vi "Adapt Class To Class.vi"() -> ()   [LabVIEW 2020]
doc: "This VI demonstrates a function of the GCraftsman JSON Serialization Toolkit.\n\nLook at the block diagram to see that the 'Adapt to Type' function adapts an object of one class type to an object of another class type. It transfers class private data values to class attributes whose names match. It successfully handles out-of-order and missing or extra class attributes \n\n'Adapt to Type' does not require the classes to have accessor methods \n\nGCraftsman JSON Object Serialization Toolkit\nwww.GCraftsman.com\nCopyright (c) 2017, GCraftsman"
uses:
  library/JKI JSON Object Serialization.lvlib
  Class2/Class2.lvclass
  Class4/Class4.lvclass
panel:
  out "class2.myBool 2":bool
  out "class2.anotherNumber 2":dbl format="%#_13g"
  out "class1.someNumber 2":dbl format="%#_13g"
  in  "class4.myBool 2":bool=TRUE
  in  "class4.someNumber 2":dbl=999.0
  in  "class4.anotherNumber 2":dbl=777.0
  out "class4.myBool":bool
  out "class4.someNumber":dbl
  out "class4.anotherNumber":dbl
  in  "class2.myBool":bool=TRUE
  in  "class2.anotherNumber":dbl=123.0 format="%#_13g"
  in  "class1.someNumber":dbl=456.0 format="%#_13g"
  # "This VI demonstrates a function of the GCraftsman JSON Serialization Toolkit.\n\nLook at the block diagram to see that the 'Adapt to Type' function adapts an object of one class type to an object of another class type.   It transfers class private data values to class attributes whose names match.  It successfully handles out-of-order and missing or extra class attributes \n \nThis example shows that 'Adapt to Type' combines heirarchical class data into a 'flat' class type, and that the 'flat' class data can successfully be distributed to private attributes in a hierarchical class structure.\n\n'Adapt to Type' does not require the classes to have accessor methods"
  # "Class 2 data"
  # "Class 4 data"
  # "parent class data"
  # "child class data"
  # "Class 4 data"
  # "Class 2 data"
  # "parent class data"
  # "child class data"
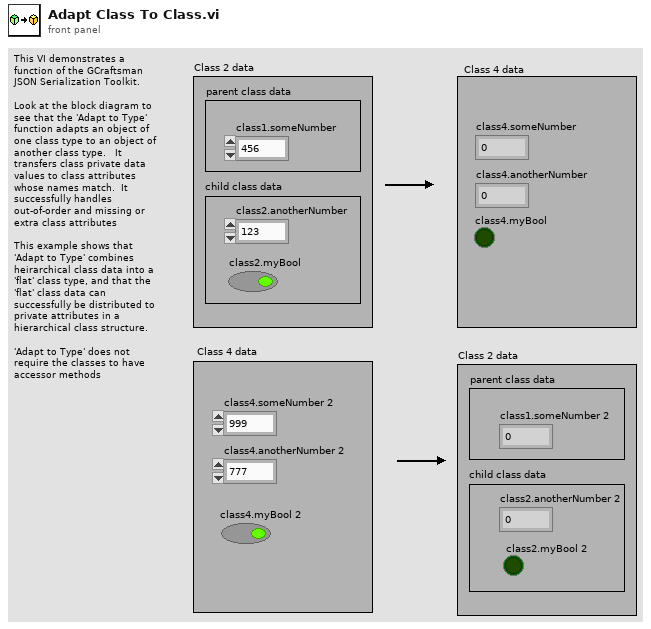
[diagram p1: front panel]
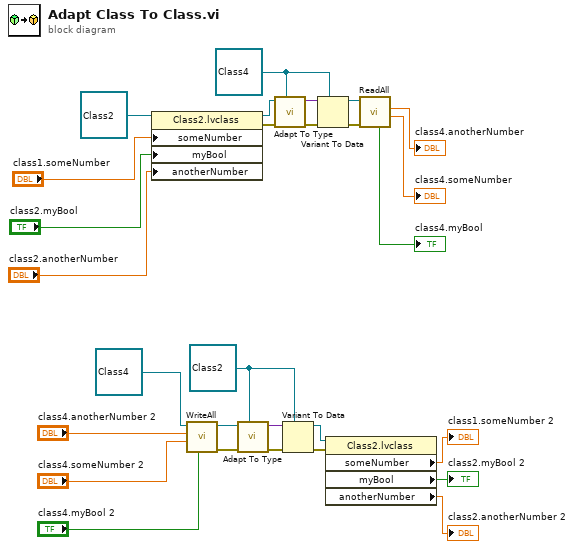
[diagram p0: block diagram]
diagram:
  w9 = refnum<class "Class2.lvclass"> refnum ("Class2.lvclass")
  w21 = refnum<class "Class4.lvclass"> refnum ("Class4.lvclass")
  n1 = property class="Class2.lvclass"(reference=refnum<class "Class2.lvclass"> refnum ("Class2.lvclass"), "someNumber"="class1.someNumber", "myBool"="class2.myBool", "anotherNumber"="class2.anotherNumber") -> (reference out=w22:refnum<class "Class2.lvclass">, error out=w18:errorcluster)  [unwired: 1 in]
  n2 = call "WriteAll.vi"("myBool"="class4.myBool 2", "someNumber"="class4.someNumber 2", "anotherNumber"="class4.anotherNumber 2", "Class4 in"=refnum<class "Class4.lvclass"> refnum ("Class4.lvclass")) -> ("error out"=w2:errorcluster, "Class4 out"=w10:refnum<class "Class4.lvclass">)  [unwired: 6 in]
  n3 = call "Adapt To Type.vi"("Type and Defaults"=w9, "error in (no error)"=w2, "Variant in"=w10) -> ("error out"=w14:errorcluster, "Variant out"=w3:variant)  [unwired: 7 in]
  n4 = call "Adapt To Type.vi"("Type and Defaults"=w21, "error in (no error)"=w18, "Variant in"=w22) -> ("error out"=w28:errorcluster, "Variant out"=w27:variant)  [unwired: 7 in]
  n5 = Variant To Data(error in=w14, type=w9, Variant=w3) -> (data=w8:refnum<class "Class2.lvclass">, error out=w7:errorcluster)
  n6 = Variant To Data(error in=w28, type=w21, Variant=w27) -> (data=w20:refnum<class "Class4.lvclass">, error out=w19:errorcluster)
  n7 = property class="Class2.lvclass"(reference=w8, error in=w7) -> ("someNumber"=→"class1.someNumber 2":dbl, "myBool"=→"class2.myBool 2":bool, "anotherNumber"=→"class2.anotherNumber 2":dbl)  [unwired: 2 out]
  n8 = call "ReadAll.vi"("error in (no error)"=w19, "Class4 in"=w20) -> ("someNumber"=→"class4.someNumber":dbl, "anotherNumber"=→"class4.anotherNumber":dbl, "myBool"=→"class4.myBool":bool)  [unwired: 5 in, 2 out]
